vi "main - UI.vi"() -> ()   [LabVIEW 2013]
doc: "Use this template to build a producer/consumer design pattern with events to produce queue items. Use this design pattern instead of the User Interface Event Handler pattern for user interfaces when you want to execute code asynchronously in response to an event without slowing the user interface responsiveness."
uses:
  TypeDef/DropletDisplay.ctl
  TypeDef/ConsumerQueue.ctl
  TypeDef/ConsumerEnum.ctl
  TypeDef/DisplayEnum.ctl
  TypeDef/DisplayQueue.ctl
  DB/DisplayGFVEnum.ctl
  DB/DisplayDB.ctl
  <vilib>/vision/Image Controls.llb/IMAQ Image.ctl
  DB/ConfDB.ctl
  DB/ConfEnum.ctl
  DB/DbEnum.ctl
panel:
  in  "Droplet Display":T1 {"Array" format="%#_1f"}
  in  "Detect Droplets Button":bool
  out "Image Out":T2(plugin-control)
  in  "Score":dbl=400.0
  in  "Temperature File Name":string="parameter.xls"
  in  "Number of images for baseline":i32=15
  out "Detla t (sec)":i32=2
  in  "N times sigam (tol)":i32=20
  in  "Number of images to save around freeze point":i32=10
  in  "End Index":i32=2187
  in  "File Path":path=path "Z:/Downloads/Fridge Pictures/1"
  in  "Start Index":i32=1
  in  "Partial Image File Name":string="cameraA-nr"
  in  "stop":bool
  # "These are updated upon selection of directory"
  # "Update main droplet display from droplet database - send result through variant"
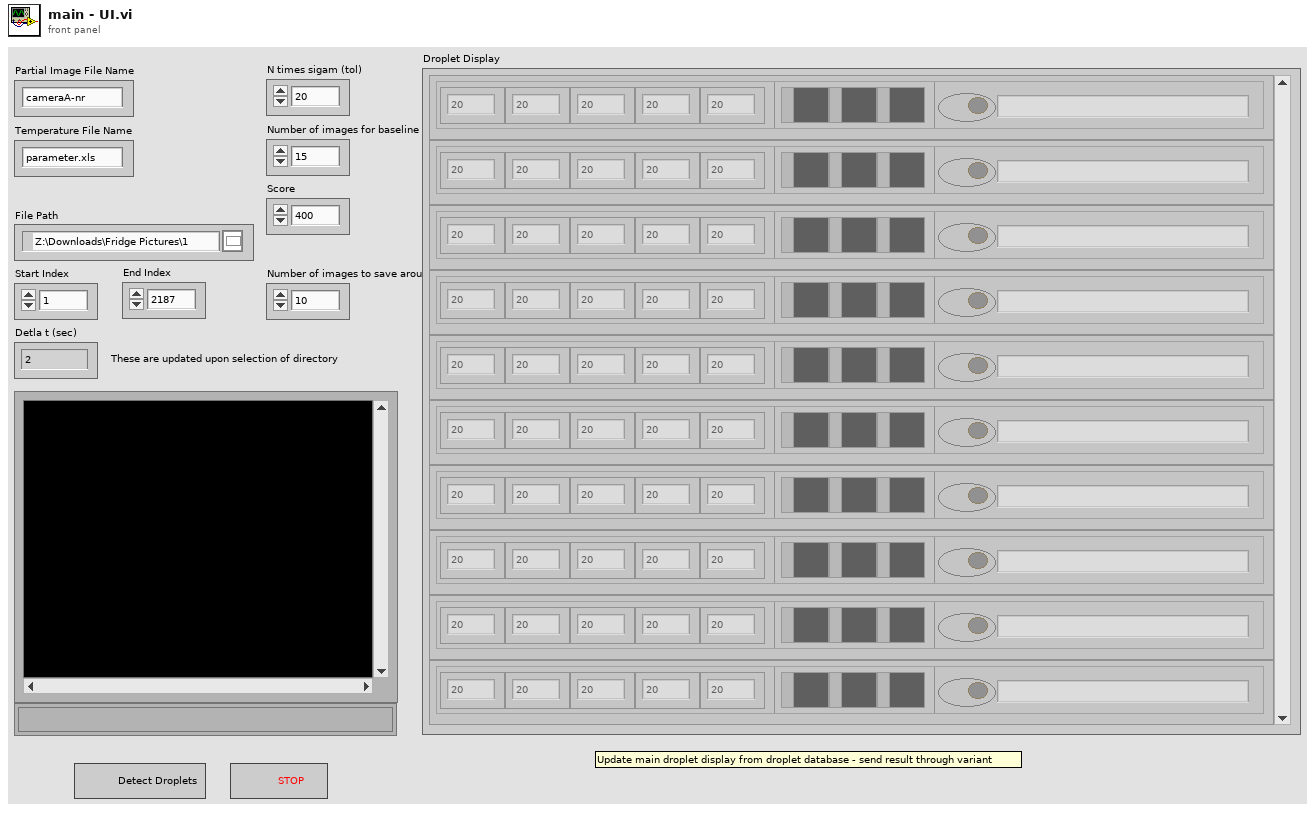
[diagram p1: front panel]
types:
  T1 = typedef "DropletDisplay.ctl" = cluster{"Array":dbl[], "Array 2":T2[], "Include Droplet":bool, "Remark":string}[]
  T2 = typedef "IMAQ Image.ctl" = refnum<image>
  T3 = typedef "DisplayQueue.ctl" = cluster{"Enum":T4, "Variant":variant}
  T4 = typedef "DisplayEnum.ctl" = enum16{"Stop Display", "Update Display", "Init Display"}
  T5 = typedef "ConsumerEnum.ctl" = enum16{"Init Configuration DB", "Init Droplet DB", "Stop", "Detect Droplets"}
  T6 = typedef "ConsumerQueue.ctl" = cluster{"Enum":T5, "Variant":variant}
  T7 = typedef "ConfEnum.ctl" = enum16{"Init", "GetConfDB", "Configure DB"}
  T8 = typedef "ConfDB.ctl" = cluster{"NumberOfImages":i32, "NoImages2SaveAroundFreeze":i32, "Path":path, "NameOfPartialFile":string, "StartIndex":i32, "NumberOfStdTol":i32, "Detla t (sec)":i32, "Number of images for baseline":i32, "Temperature File Name":string, "Score":dbl, "Index number of Files":i32[]}
  T9 = typedef "DisplayGFVEnum.ctl" = enum16{"Update Display", "Get Image Ref", "Insert Image Ref to Display", "Init Display"}
  T10 = typedef "DbEnum.ctl" = enum16{"Init", "Insert Detection Result Data", "Insert Grey Level Result", "Insert Baseline Results", "Insert Freeze Analysis Results", "GetDropDB", "GetDropletsBoundingBox"}
  T11 = cluster{"Position":cluster{"x":sgl, "y":sgl}, "Angle":sgl, "Scale":sgl, "Score":sgl, "Bounding Box":cluster{"x":sgl, "y":sgl}[]}[]
  T12 = typedef "DisplayDB.ctl" = cluster{"Image Ref":T2}
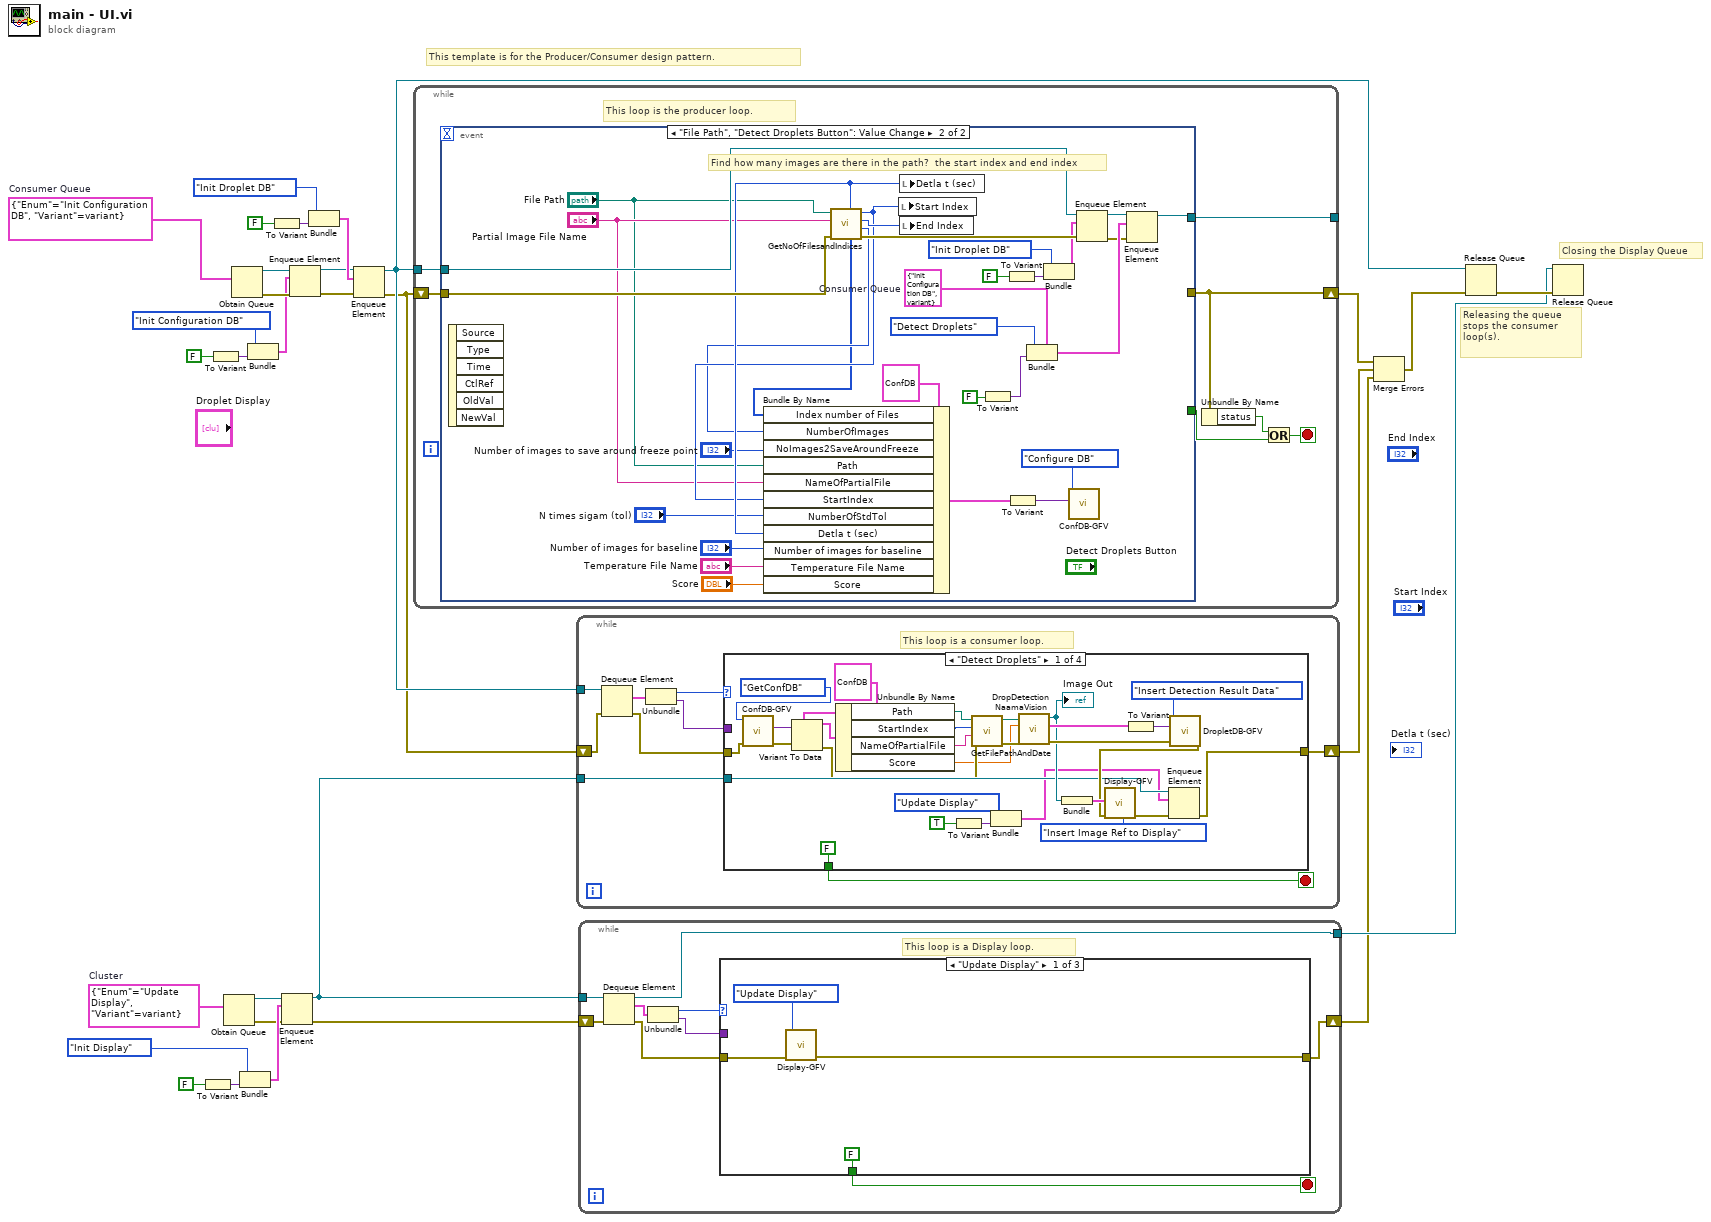
[diagram p0: block diagram]
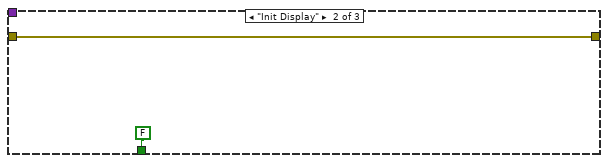
[diagram p2: hidden frame]
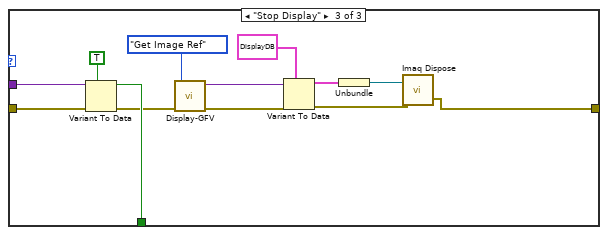
[diagram p3: hidden frame]
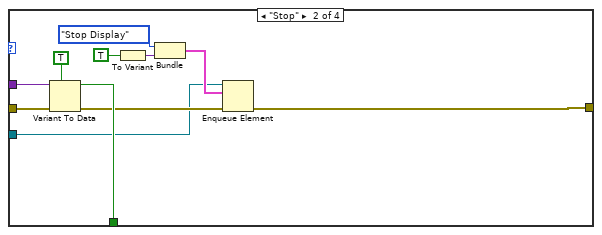
[diagram p4: hidden frame]
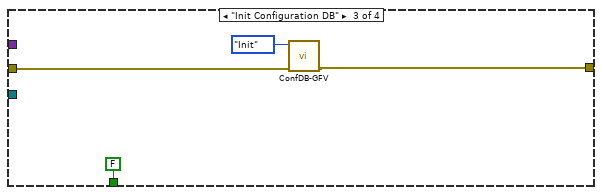
[diagram p5: hidden frame]
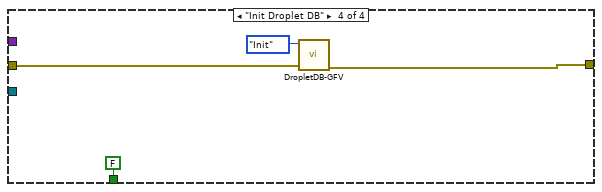
[diagram p6: hidden frame]
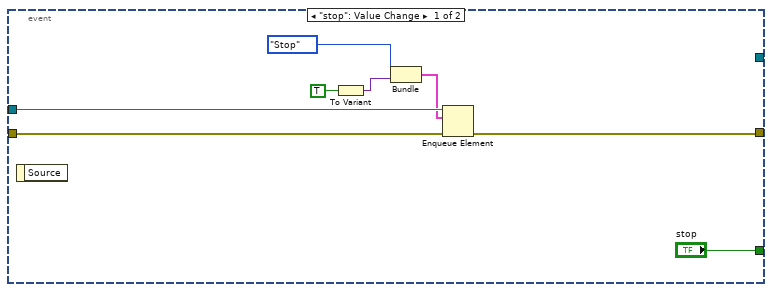
[diagram p7: hidden frame]
diagram:
  w6 = T3 {"Enum"=enum."Update Display", "Variant"=variant}  # Cluster
  w30 = T6 {"Enum"=enum."Init Configuration DB", "Variant"=variant}  # Consumer Queue
  # "Closing the Display Queue"
  # "Releasing the queue stops the consumer loop(s)."
  # "This template is for the Producer/Consumer design pattern."
  n1 = To Variant(anything=FALSE) -> (Variant=w11:variant)
  n2 = To Variant(anything=FALSE) -> (Variant=w15:variant)
  n3 = Obtain Queue(element data type=w6) -> (queue out=w8:refnum<queue>, error out=w9:errorcluster)  [unwired: 4 in, 1 out]
  n4 = Obtain Queue(element data type=w30) -> (queue out=w20:refnum<queue>, error out=w19:errorcluster)  [unwired: 4 in, 1 out]
  n5 = Bundle("Enum"=DisplayEnum."Init Display", "Variant"=w11) -> (w12:cluster{"Enum":T4, "Variant":variant})  [unwired: 1 in]
  n6 = Bundle(ConsumerEnum."Init Configuration DB", "Variant"=w15) -> (w13:cluster{T5, "Variant":variant})  [unwired: 1 in]
  n7 = To Variant(anything=FALSE) -> (Variant=w22:variant)
  n8 = Enqueue Element(queue=w8, element=w12, error in (no error)=w9) -> (queue out=w5:refnum<queue>, error out=w4:errorcluster)  [unwired: 1 in, 1 out]
  n9 = Enqueue Element(queue=w20, element=w13, error in (no error)=w19) -> (queue out=w17:refnum<queue>, error out=w18:errorcluster)  [unwired: 1 in, 1 out]
  n10 = Bundle(ConsumerEnum."Init Droplet DB", "Variant"=w22) -> (w23:cluster{T5, "Variant":variant})  [unwired: 1 in]
  n11 = Enqueue Element(queue=w17, element=w23, error in (no error)=w18) -> (queue out=w26:refnum<queue>, error out=w25:errorcluster)  [unwired: 1 in, 1 out]
  n12 = while {
    shift-right: [w33] -> w29
    shift-left: w25 -> [w36]
    tunnel: w26 -> [w37]
    tunnel: [w31] -> _
    stop <- w34 stop-if-true
    # "This loop is the producer loop."
    n13 = event shown="[1] \"File Path\", \"Detect Droplets Button\": Value Change" {
      selector: _ -> [_ _]
      dyn-events: _ -> [_ _]
      timeout: _ -> [_ _]
      tunnel: w37 -> [w44 w69]
      tunnel: w36 -> [w43 w76]
      tunnel: [w42 _] -> w33
      tunnel: ["stop" _] -> w35
      tunnel: [_ w71] -> w31
      event "stop": Value Change {
        n14 = event-data() -> ()  [unwired: 1 in, 1 out]
        n15 = To Variant(anything=TRUE) -> (Variant=w39:variant)
        n16 = Bundle(ConsumerEnum."Stop", "Variant"=w39) -> (w38:cluster{T5, "Variant":variant})  [unwired: 1 in]
        n17 = Enqueue Element(queue=w44, element=w38, error in (no error)=w43) -> (error out=w42:errorcluster)  [unwired: 1 in, 2 out]
      }
      event "File Path", "Detect Droplets Button": Value Change {
        w73 = T6 {"Enum"=enum."Init Configuration DB", "Variant"=variant}  # Consumer Queue
        # "Find how many images are there in the path?  the start index and end index"
        n18 = event-data() -> ()  [unwired: 1 in, 6 out]
        n19 = call "GetNoOfFilesandIndices.vi"("error in (no error)"=w76, "Partial Image File Name"="Partial Image File Name", "File Path"="File Path") -> ("error out"=w67:errorcluster, "Number of Files"=w50:i32, "max value"=w75:i32, "min value"=w53:i32, "Index number of Files"=w48:i32[], "Dt"=w55:u32)  [unwired: 3 in]
        n20 = Bundle By Name(cluster=T8 {"NumberOfImages"=0, "NoImages2SaveAroundFreeze"=0, "Path"=path "", "NameOfPartialFile"="", "StartIndex"=0, "NumberOfStdTol"=0, "Detla t (sec)"=0, "Number of images for baseline"=0, "Temperature File Name"="", "Score"=0.0, "Index number of Files"=[]} ("ConfDB"), "Index number of Files"=w48, "NumberOfImages"=w50, "NoImages2SaveAroundFreeze"="Number of images to save around freeze point", "Path"="File Path", "NameOfPartialFile"="Partial Image File Name", "StartIndex"=w53, "NumberOfStdTol"="N times sigam (tol)", "Detla t (sec)"=w55, "Number of images for baseline"="Number of images for baseline", "Temperature File Name"="Temperature File Name", "Score"="Score") -> (w59:T8)
        n21 = local write "Start Index"(w53) -> ()
        n22 = local write "Detla t (sec)"(w55) -> ()
        n23 = local write "End Index"(w75) -> ()
        n24 = To Variant(anything=FALSE) -> (Variant=w70:variant)
        n25 = To Variant(anything=FALSE) -> (Variant=w64:variant)
        n26 = To Variant(anything=w59) -> (Variant=w60:variant)
        n27 = Bundle(cluster=w73, "Enum"=ConsumerEnum."Detect Droplets", "Variant"=w70) -> (w72:T6)
        n28 = Bundle(ConsumerEnum."Init Droplet DB", "Variant"=w64) -> (w62:cluster{T5, "Variant":variant})  [unwired: 1 in]
        n29 = call "ConfDB-GFV.vi"("Data in"=w60, "Command In"=ConfEnum."Configure DB") -> ()  [unwired: 8 in, 2 out]
        n30 = Enqueue Element(queue=w69, element=w62, error in (no error)=w67) -> (queue out=w68:refnum<queue>, error out=w66:errorcluster)  [unwired: 1 in, 1 out]
        n31 = Enqueue Element(queue=w68, element=w72, error in (no error)=w66) -> (queue out=w71:refnum<queue>)  [unwired: 1 in, 2 out]
      }
    }
    n32 = Unbundle By Name(w33) -> ("status"=w32:bool)
    n33 = Or(x=w32, y=w35) -> (x .or. y?=w34:bool)
  }
  n34 = while {
    tunnel: w26 -> [w85]
    shift-right: [w79] -> w28
    shift-left: w25 -> [w81]
    tunnel: w5 -> [w77]
    stop <- w78 stop-if-true
    # "This loop is a consumer loop."
    n35 = Dequeue Element(queue=w85, error in (no error)=w81) -> (element=w84:T6, error out=w80:errorcluster)  [unwired: 1 in, 2 out]
    n36 = Unbundle(w84) -> ("Enum"=w83:T5, "Variant"=w82:variant)
    n37 = case shown="\"Detect Droplets\"" w83 {
      tunnel: w82 -> [_ w124 _ _]
      tunnel: w80 -> [w95 w125 w127 w132]
      tunnel: [w97 w120 w126 w131] -> w79
      tunnel: [FALSE w122 FALSE FALSE] -> w78
      tunnel: w77 -> [w103 w115 _ _]
      frame "Detect Droplets" {
        n38 = call "ConfDB-GFV.vi"("error in (no error)"=w95, "Command In"=ConfEnum."GetConfDB") -> ("error out"=w92:errorcluster, "Data out"=w94:variant)  [unwired: 8 in]
        n39 = Variant To Data(error in=w92, type=T8 {"NumberOfImages"=0, "NoImages2SaveAroundFreeze"=0, "Path"=path "", "NameOfPartialFile"="", "StartIndex"=0, "NumberOfStdTol"=0, "Detla t (sec)"=0, "Number of images for baseline"=0, "Temperature File Name"="", "Score"=0.0, "Index number of Files"=[]} ("ConfDB"), Variant=w94) -> (data=w90:T8, error out=w91:errorcluster)
        n40 = Unbundle By Name(w90) -> ("Path"=w89:path, "StartIndex"=w88:i32, "NameOfPartialFile"=w87:string, "Score"=w86:dbl)
        n41 = To Variant(anything=TRUE) -> (Variant=w101:variant)
        n42 = call "GetFilePathAndDate.vi"("error in (no error)"=w91, "String"=w87, "Index"=w88, "Path"=w89) -> ("error out"=w114:errorcluster, "file out"=w113:path)  [unwired: 5 in, 1 out]
        n43 = Bundle("Enum"=DisplayEnum."Update Display", "Variant"=w101) -> (w99:cluster{"Enum":T4, "Variant":variant})  [unwired: 1 in]
        n44 = call "DropDetection NaamaVision.vi"("error in"=w114, "Minimum Match Score"=w86, "Path"=w113) -> ("error out"=w109:errorcluster, "Matches (pixel)"=w108:T11, "Image Out"=w106:T2)  [unwired: 5 in, 1 out]
        "Image Out" <- w106
        n45 = Bundle("Image Out"=w106) -> (w105:cluster{"Image Out":T2})  [unwired: 1 in]
        n46 = To Variant(anything=w108) -> (Variant=w111:variant)
        n47 = call "DropletDB-GFV.vi"("error in (no error)"=w109, "Data in"=w111, "Command In"=DbEnum."Insert Detection Result Data") -> ("error out"=w104:errorcluster)  [unwired: 7 in, 1 out]
        n48 = call "Display-GFV.vi"("error in (no error)"=w104, "Data in"=w105, 11:DisplayGFVEnum."Insert Image Ref to Display") -> ("error out"=w98:errorcluster)  [unwired: 7 in, 1 out]
        n49 = Enqueue Element(queue=w103, element=w99, error in (no error)=w98) -> (error out=w97:errorcluster)  [unwired: 1 in, 2 out]
      }
      frame "Stop" {
        n50 = Variant To Data(error in=w125, type=TRUE, Variant=w124) -> (data=w122:bool, error out=w121:errorcluster)
        n51 = To Variant(anything=TRUE) -> (Variant=w118:variant)
        n52 = Bundle("Enum"=DisplayEnum."Stop Display", "Variant"=w118) -> (w116:cluster{"Enum":T4, "Variant":variant})  [unwired: 1 in]
        n53 = Enqueue Element(queue=w115, element=w116, error in (no error)=w121) -> (error out=w120:errorcluster)  [unwired: 1 in, 2 out]
      }
      frame "Init Configuration DB" {
        n54 = call "ConfDB-GFV.vi"("error in (no error)"=w127, "Command In"=ConfEnum."Init" ("Command")) -> ("error out"=w126:errorcluster)  [unwired: 8 in, 1 out]
      }
      frame "Init Droplet DB" {
        n55 = call "DropletDB-GFV.vi"("error in (no error)"=w132, "Command In"=DbEnum."Init") -> ("error out"=w131:errorcluster)  [unwired: 8 in, 1 out]
      }
    }
  }
  n56 = while {
    shift-right: [w134] -> w1
    shift-left: w4 -> [w140]
    tunnel: w5 -> [w137]
    tunnel: [w135] -> w2
    stop <- w138 stop-if-true
    # "This loop is a Display loop."
    n57 = Dequeue Element(queue=w137, error in (no error)=w140) -> (queue out=w135:refnum<queue>, element=w142:T3, error out=w139:errorcluster)  [unwired: 1 in, 1 out]
    n58 = Unbundle(w142) -> ("Enum"=w136:T4, "Variant"=w141:variant)
    n59 = case shown="\"Update Display\"" w136 {
      tunnel: w141 -> [_ _ w159]
      tunnel: w139 -> [w144 w147 w160]
      tunnel: [FALSE FALSE w158] -> w138
      tunnel: [w143 w147 w149] -> w134
      frame "Update Display" {
        n60 = call "Display-GFV.vi"("error in (no error)"=w144, 11:DisplayGFVEnum."Update Display") -> ("error out"=w143:errorcluster)  [unwired: 8 in, 1 out]
      }
      frame "Init Display" {
      }
      frame "Stop Display" {
        n61 = Variant To Data(error in=w160, type=TRUE, Variant=w159) -> (data=w158:bool, error out=w157:errorcluster)
        n62 = call "Display-GFV.vi"("error in (no error)"=w157, 11:DisplayGFVEnum."Get Image Ref") -> ("error out"=w155:errorcluster, "Data out"=w154:variant)  [unwired: 8 in]
        n63 = Variant To Data(error in=w155, type=T12 {"Image Ref"=refnum} ("Display Cluster"), Variant=w154) -> (data=w152:T12, error out=w150:errorcluster)
        n64 = Unbundle(w152) -> ("Image Ref"=w151:T2)
        n65 = call "Imaq Dispose"("Image"=w151, "error in (no error)"=w150) -> ("error out"=w149:errorcluster)  [unwired: 4 in]
      }
    }
  }
  n66 = Merge Errors(w29, w28, w1) -> (w27:errorcluster)
  n67 = Release Queue(queue=w26, error in (no error)=w27) -> (error out=w3:errorcluster)  [unwired: 1 in, 2 out]
  n68 = Release Queue(queue=w2, error in (no error)=w3) -> ()  [unwired: 1 in, 3 out]
